vi "Stuff Cluster.vi"(11 "output cluster":T1) -> (3 "reference out":refnum<vi>)   [LabVIEW 2016]
uses:
  Controls/Cal Refs.ctl
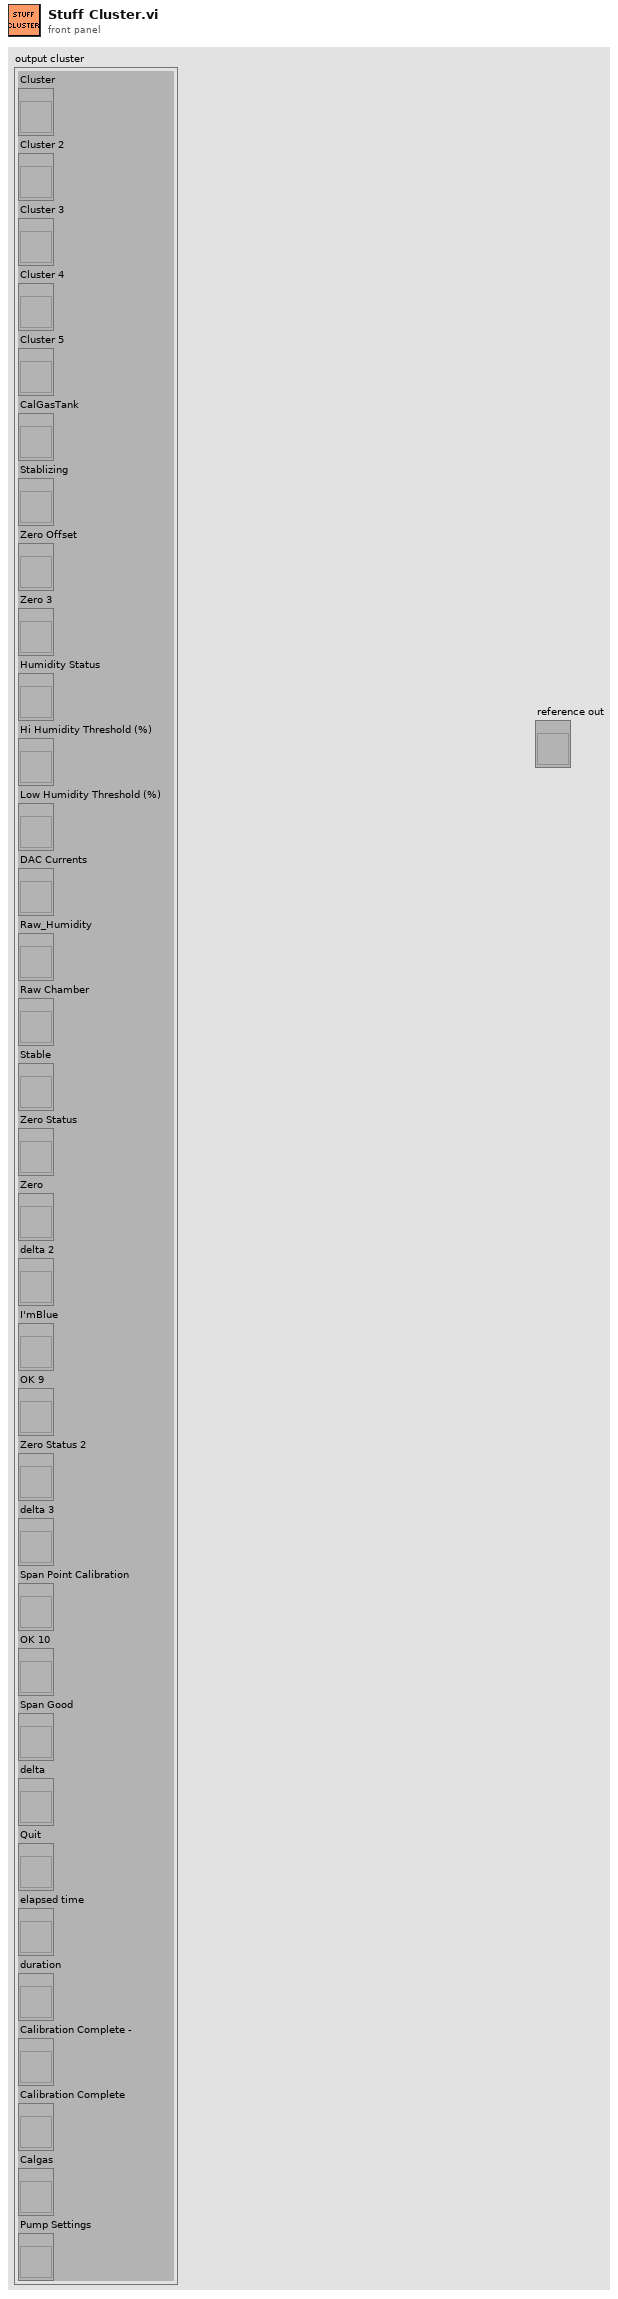
[diagram p1: front panel]
types:
  T1 = typedef "Cal Refs.ctl" = cluster{"Cluster":refnum<vi>, "Cluster 2":refnum<vi>, "Cluster 3":refnum<vi>, "Cluster 4":refnum<vi>, "Cluster 5":refnum<vi>, "CalGasTank":refnum<vi>, "Stablizing":refnum<vi>, "Zero Offset":refnum<vi>, "Zero 3":refnum<vi>, "Humidity Status":refnum<vi>, "Hi Humidity Threshold (%)":refnum<vi>, "Low Humidity Threshold (%)":refnum<vi>, "DAC Currents":refnum<vi>, "Raw_Humidity":refnum<vi>, "Raw Chamber":refnum<vi>, "Stable":refnum<vi>, "Zero Status":refnum<vi>, "Zero":refnum<vi>, "delta 2":refnum<vi>, "I'mBlue":refnum<vi>, "OK 9":refnum<vi>, "Zero Status 2":refnum<vi>, "delta 3":refnum<vi>, "Span Point Calibration":refnum<vi>, "OK 10":refnum<vi>, "Span Good":refnum<vi>, "delta":refnum<vi>, "Quit":refnum<vi>, "elapsed time":refnum<vi>, "duration":refnum<vi>, "Calibration Complete -":refnum<vi>, "Calibration Complete":refnum<vi>, "Calgas":refnum<vi>, "Pump Settings":refnum<vi>}
  T2 = cluster{"Tcal_Chamber":dbl, "Tcal_PCB":dbl, "Tcal_Film":dbl, "Tcal_Humidity":dbl, "Tcal_Det":dbl[], "Cal Gas":dbl, "Reference":dbl}
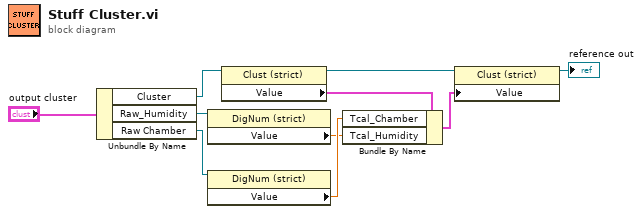
[diagram p0: block diagram]
diagram:
  n1 = Unbundle By Name("output cluster") -> ("Cluster"=w6:refnum<vi>, "Raw_Humidity"=w7:refnum<vi>, "Raw Chamber"=w9:refnum<vi>)
  n2 = property class="DigNum (strict)"(reference=w7) -> ("Value"=w8:dbl)  [unwired: 1 in, 2 out]
  n3 = property class="DigNum (strict)"(reference=w9) -> ("Value"=w10:dbl)  [unwired: 1 in, 2 out]
  n4 = property class="Clust (strict)"(reference=w6) -> (reference out=w2:refnum<vi>, "Value"=w3:T2)  [unwired: 1 in, 1 out]
  n5 = Bundle By Name(cluster=w3, "Tcal_Chamber"=w10, "Tcal_Humidity"=w8) -> (w4:T2)
  n6 = property class="Clust (strict)"(reference=w2, "Value"=w4) -> (reference out=→"reference out":refnum<vi>)  [unwired: 1 in, 1 out]
